vi "Remove Shared Memory File.vi"(8 "error in (no error)":errorcluster, 11 "shared memory in":T1) -> (0 "error out":errorcluster, 3 "shared memory name":string)   [LabVIEW 2013, in "Linux RT IPC.lvlib" / "Shared Memory.lvlib" / "Shared Memory.lvclass"]
doc: "This VI unlinks from the shared memory file. If other processes are linked to the shared memory, their memory mapping will remain. However, the shared memory file will be removed from the filesystem, preventing new mappings from being made."
uses:
  Shared Memory.lvclass
  Controls/reference.ctl
  Shared Memory.lvclass/Shared Memory.ctl
  C/C.lvlib
  Shared Memory.lvlib
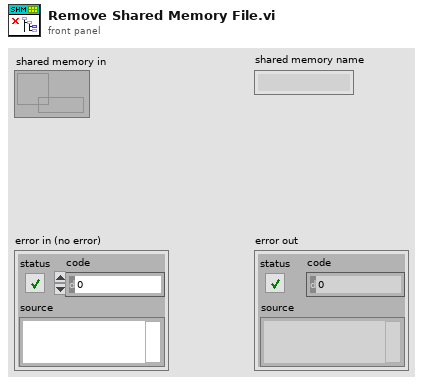
[diagram p1: front panel]
types:
  T1 = typedef "Linux RT IPC.lvlib/Shared Memory.lvlib/reference.ctl" = refnum<data-value>
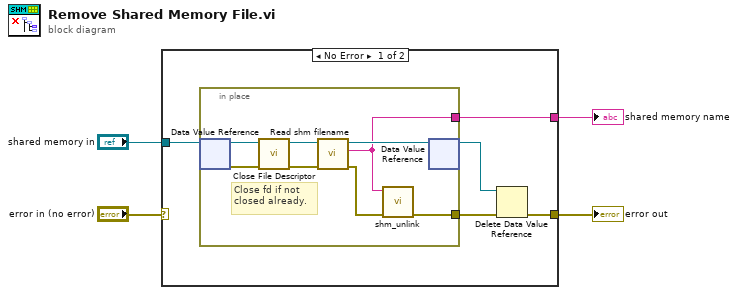
[diagram p0: block diagram]
diagram:
  n1 = case shown="No Error" "error in (no error)" {
    selector: "error in (no error)" -> [_ w18]
    tunnel: "shared memory in" -> [w9 _]
    tunnel: [w6 w18] -> w2
    tunnel: [w8 _] -> w1
    frame No Error {
      n2 = in-place {
        in-place-border: [w10] -> w7
        in-place-border: [w11] -> w8
        # "Close fd if not closed already."
        n3 = in-place-dvr #1(w9) -> (w17:refnum<class "Shared Memory.lvclass">, w16:errorcluster)
        n4 = call "Close File Descriptor.vi"("error in (no error)"=w16, "Shared Memory in"=w17) -> ("error out"=w13:errorcluster, "Shared Memory out"=w14:refnum<class "Shared Memory.lvclass">)  [unwired: 8 in]
        n5 = call "Read shm filename.vi"("error in (no error)"=w13, "Shared Memory in"=w14) -> ("error out"=w15:errorcluster, "shm filename"=w11:string, "Shared Memory out"=w12:refnum<class "Shared Memory.lvclass">)  [unwired: 7 in]
        n6 = call "shm_unlink.vi"("error in (no error)"=w15, "name"=w11) -> ("error out"=w10:errorcluster)  [unwired: 9 in]
        n7 = in-place-dvr #1(w12) -> (w5:T1)  [unwired: 1 out]
      }
      n8 = Delete Data Value Reference(data value reference=w5, error in=w7) -> (error out=w6:errorcluster)  [unwired: 1 out]
    }
    frame Error {
    }
  }
  "error out" <- w2
  "shared memory name" <- w1
